vi "CC Script Parse Pause.vi"(8 "error in (no error)":errorcluster, 11 "DefineObject Parameters":string="(11.000000)") -> (0 "error out":errorcluster, 3 "Pause Parameters":T1)   [LabVIEW 2021]
uses:
  typedefs/CC cluster Pause Parameters.ctl
  <vilib>/regexp/Match Regular Expression.xnode
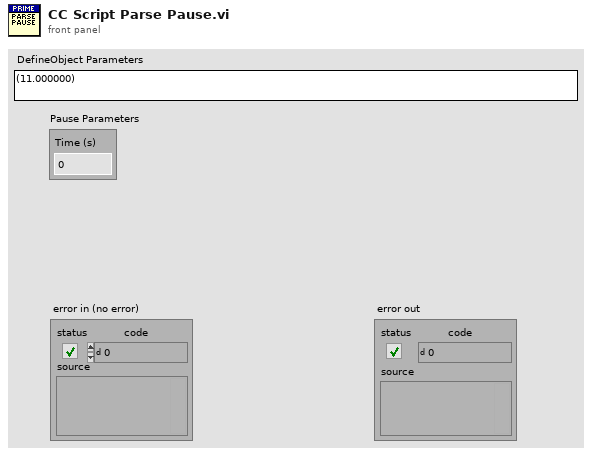
[diagram p1: front panel]
types:
  T1 = typedef "CC cluster Pause Parameters.ctl" = cluster{"Time (s)":dbl}
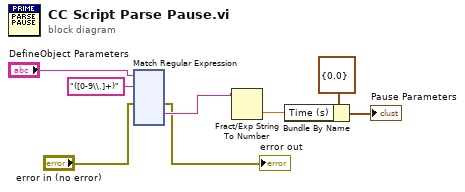
[diagram p0: block diagram]
diagram:
  n1 = xnode "Match Regular Expression"("input string"="DefineObject Parameters", "regular expression"="([0-9\\.]+)", "error in"="error in (no error)") -> ("error out"=→"error out":errorcluster, "submatch 1"=w5:string)  [unwired: 3 in, 5 out]
  n2 = Fract/Exp String To Number(string=w5) -> (number=w4:dbl)  [unwired: 3 in, 1 out]
  n3 = Bundle By Name(cluster=T1 {"Time (s)"=0.0} ("Pause Parameters"), "Time (s)"=w4) -> (→"Pause Parameters":T1)
